vi "Start Executor.vi"(8 "error in (no error)":errorcluster, 9 "Semaphore":T1, 10 "Value":variant, 11 "Callbacks":refnum<queue>) -> ()   [LabVIEW 2017, in "Promise Future.lvlib" / "State.lvclass"]
uses:
  State.lvclass
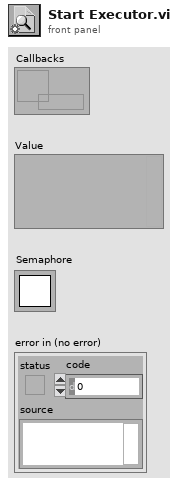
[diagram p1: front panel]
types:
  T1 = typedef "Semaphore RefNum" = refnum<k1>
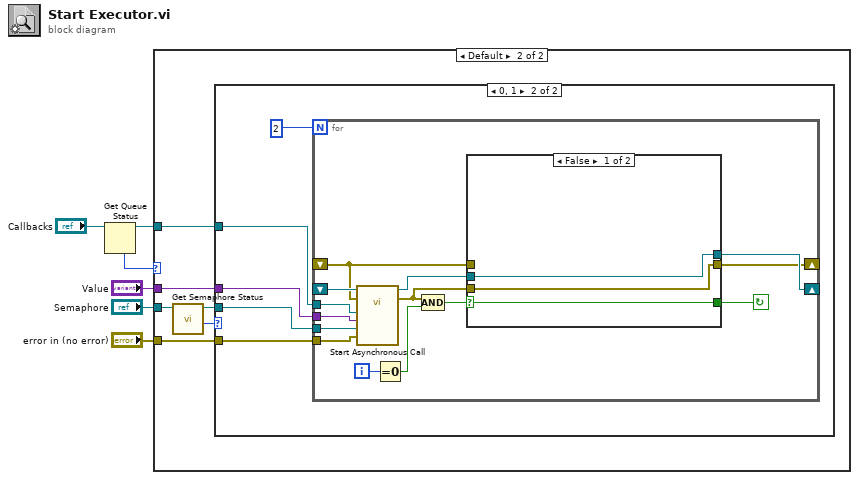
[diagram p0: block diagram]
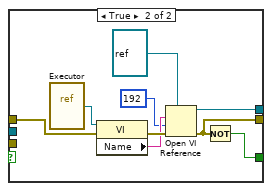
[diagram p4: hidden frame]
diagram:
  n1 = Get Queue Status(queue="Callbacks") -> (queue out=w4:refnum<queue>, # elements in queue=w5:i32)  [unwired: 2 in, 6 out]
  n2 = case shown="Default" w5 {
    tunnel: "Semaphore" -> [_ w11]
    tunnel: w4 -> [_ w10]
    tunnel: "Value" -> [_ w9]
    tunnel: "error in (no error)" -> [_ w7]
    frame 0 {
      # "No waiting callbacks, no need for an executor"
    }
    frame Default {
      n3 = call <vilib>:"Get Semaphore Status.vi"("semaphore"=w11) -> ("# waiting"=w12:i32, "semaphore out"=w8:T1)  [unwired: 5 in, 4 out]
      n4 = case shown="0, 1" w12 {
        tunnel: w10 -> [_ w16]
        tunnel: w9 -> [_ w15]
        tunnel: w8 -> [_ w14]
        tunnel: w7 -> [_ w13]
        frame Default {
          # "Already have another executor waiting for the queue, don't bother launching more"
        }
        frame 0, 1 {
          n5 = for {
            N: 2 -> [_]
            shift-right: [w31] -> _
            shift-left: _ -> [w23]
            shift-right: [w30] -> _
            shift-left: _ -> [w22]
            tunnel: w16 -> [w21]
            tunnel: w15 -> [w20]
            tunnel: w14 -> [w19]
            tunnel: w13 -> [w18]
            i -> [w27]
            stop <- w26 continue-if-true
            n6 = call-by-ref "Start Asynchronous Call"(reference=w23, error in=w22, 8:"error in (no error)"=w18, "semaphore"=w19, "Value"=w20, "Callbacks"=w21) -> (reference out=w25:refnum<vi>, error out=w24:errorcluster)  [unwired: 8 in]
            n7 = Equal To 0?(x=w27) -> (x = 0?=w28:bool)
            n8 = Compound Arithmetic op=AND(w24, w28) -> (w29:bool)
            n9 = case shown="False" w29 {
              selector: w29 -> [w32 _]
              tunnel: [w34 w40] -> w31
              tunnel: [w33 w38] -> w30
              tunnel: w25 -> [w34 _]
              tunnel: w24 -> [w33 _]
              tunnel: [w32 w39] -> w26
              tunnel: w22 -> [_ w37]
              frame False {
              }
              frame True {
                n10 = vi-ref "Executor.vi"() -> (w36:refnum<vi>)
                n11 = property class="VI"(reference=w36, error in=w37) -> (error out=w43:errorcluster, "Name"=w42:string)  [unwired: 1 out]
                n12 = Open VI Reference(type specifier VI Refnum (for type only)=refnum<vi> refnum, vi path=w42, options=192, error in (no error)=w43) -> (vi reference=w40:refnum<vi>, error out=w38:errorcluster)  [unwired: 2 in]
                n13 = Not(x=w38) -> (.not. x?=w39:bool)
              }
            }
          }
        }
      }
    }
  }
